vi "Program06.vi"() -> ()   [LabVIEW 2020]
panel:
  out "Po FB":dbl
  out "Przed FB":dbl
  out "Wynik":dbl[](array[numeric])
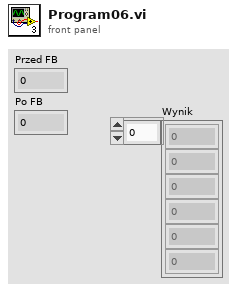
[diagram p1: front panel]
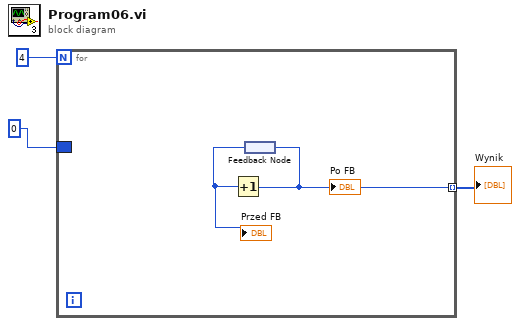
[diagram p0: block diagram]
diagram:
  n1 = for {
    N: 4 -> [_]
    border: 0 -> [_]
    tunnel: [w4] -> w1 mode=indexing
    n2 = feedback #1() -> (w5:i32)
    "Przed FB" <- w5
    n3 = Increment(x=w5) -> (x+1=w4:i32)
    "Po FB" <- w4
    n4 = feedback-in #1(w4) -> ()
  }
  "Wynik" <- w1
